vi "GetAllAxisPositions.vi"(8 "error in (no error)":errorcluster, 11 "Picomoto8742ControllerClass in":refnum<class "Picomoto8742ControllerClass.lvclass">) -> (0 "error out":errorcluster, 2 "AxisPositions":i32[](array[numeric]), 3 "Picomoto8742ControllerClass out":refnum<class "Picomoto8742ControllerClass.lvclass">)   [LabVIEW 2013, in "Picomoto8742ControllerClass.lvclass"]
doc: "Query all the axis positions from the physical device"
uses:
  Picomoto8742ControllerClass.lvclass
  Picomoto8742ControllerClass.lvclass/Picomoto8742ControllerClass.ctl
  PicoMotor8742Axis/Picomotor8742Axis.lvclass
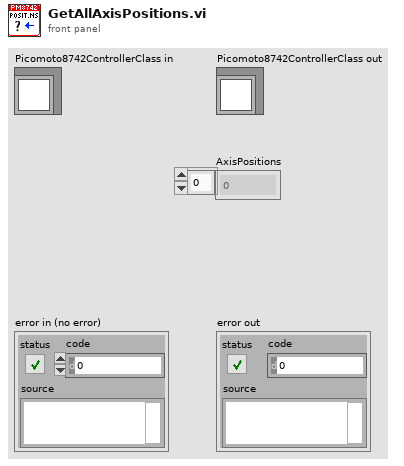
[diagram p1: front panel]
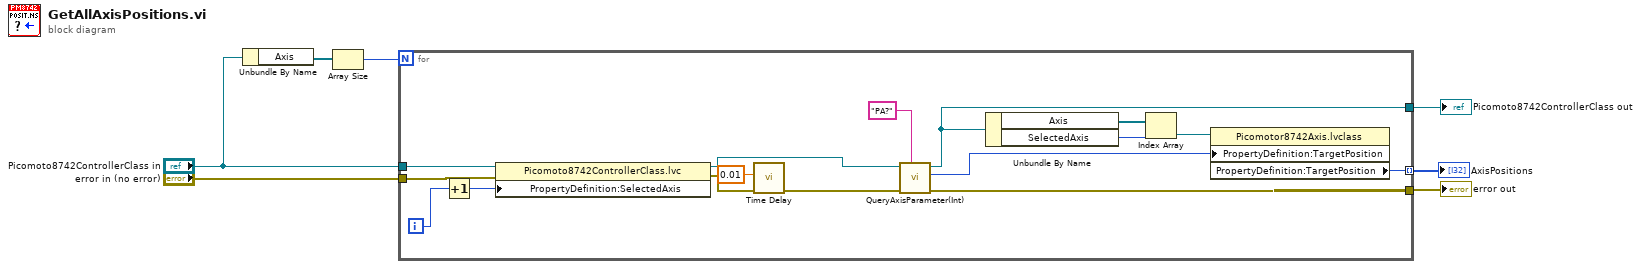
[diagram p0: block diagram]
diagram:
  n1 = Unbundle By Name("Picomoto8742ControllerClass in") -> ("Axis"=w4:refnum<class "Picomotor8742Axis.lvclass">[])
  n2 = Array Size(array=w4) -> (size(s)=w3:i32)
  n3 = for {
    N: w3 -> [_]
    tunnel: "Picomoto8742ControllerClass in" -> [w23]
    tunnel: [w17] -> w6
    tunnel: "error in (no error)" -> [w16]
    tunnel: [w10] -> w1 mode=indexing
    tunnel: [w9] -> w2
    i -> [w14]
    n4 = Increment(x=w14) -> (x+1=w22:i32)
    n5 = property class="Picomoto8742ControllerClass.lvc"(reference=w23, error in=w16, "PropertyDefinition:SelectedAxis"=w22) -> (reference out=w20:refnum<class "Picomoto8742ControllerClass.lvclass">, error out=w19:errorcluster)
    n6 = call "Time Delay"("error in (no error)"=w19, "Delay Time (s)"=0.01) -> ("error out"=w18:errorcluster)  [unwired: 9 in]
    n7 = call-dynamic "QueryAxisParameter(Int).vi"("Cmd"="PA?" ("string"), "error in (no error)"=w18, "Picomoto8742ControllerClass in"=w20) -> ("error out"=w17:errorcluster, "ValueOut"=w11:i32, "Picomoto8742ControllerClass Out"=w9:refnum<class "Picomoto8742ControllerClass.lvclass">)  [unwired: 6 in]
    n8 = Unbundle By Name(w9) -> ("Axis"=w15:refnum<class "Picomotor8742Axis.lvclass">[], "SelectedAxis"=w13:u32)
    n9 = Index Array(array=w15, index=w13) -> (element=w12:refnum<class "Picomotor8742Axis.lvclass">)
    n10 = property class="Picomotor8742Axis.lvclass"(reference=w12, "PropertyDefinition:TargetPosition"=w11) -> ("PropertyDefinition:TargetPosition"=w10:i32)  [unwired: 1 in, 2 out]
  }
  "error out" <- w6
  "Picomoto8742ControllerClass out" <- w2
  "AxisPositions" <- w1
